vi "Tracker_hardware_setup.vi"(0 "VISA resource name":refnum<visa-resource-name>="ASRL3::INSTR", 2 "Close port? (T)":bool) -> (6 "error out":errorcluster, 7 "VISA resource name out":refnum<visa-resource-name>, 8 "ReadStatus":refnum<notifier>, 9 "error":bool, 10 "Record_flag":refnum<notifier>)   [LabVIEW 2016]
uses:
  <vilib>/Instr/_visa.llb/VISA Set IO Buffer Mask.ctl
  <vilib>/Instr/_visa.llb/VISA Configure Serial Port (Instr).vi
  Globaltracker.vi
panel:
  out "Poll Port data status":u32
  out "Port data status":i32
  out "error out 2":errorcluster
  out "read buffer":string
  out "Poll Binary":u32
  out "Poll Matrix":u32
  out "Poll Coord":u32
  out "Poll FPS":u32
  out "FPS status":i32
  out "Matrix mode status":string
  out "Coordinate mode status":string
  out "Binary mode status":string
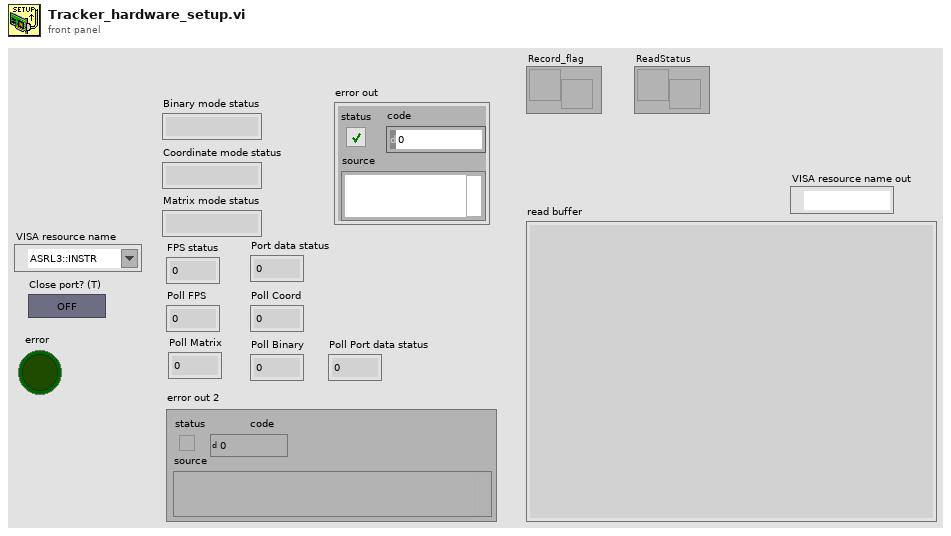
[diagram p1: front panel]
types:
  T1 = typedef "VISA Set IO Buffer Mask.ctl" = u16
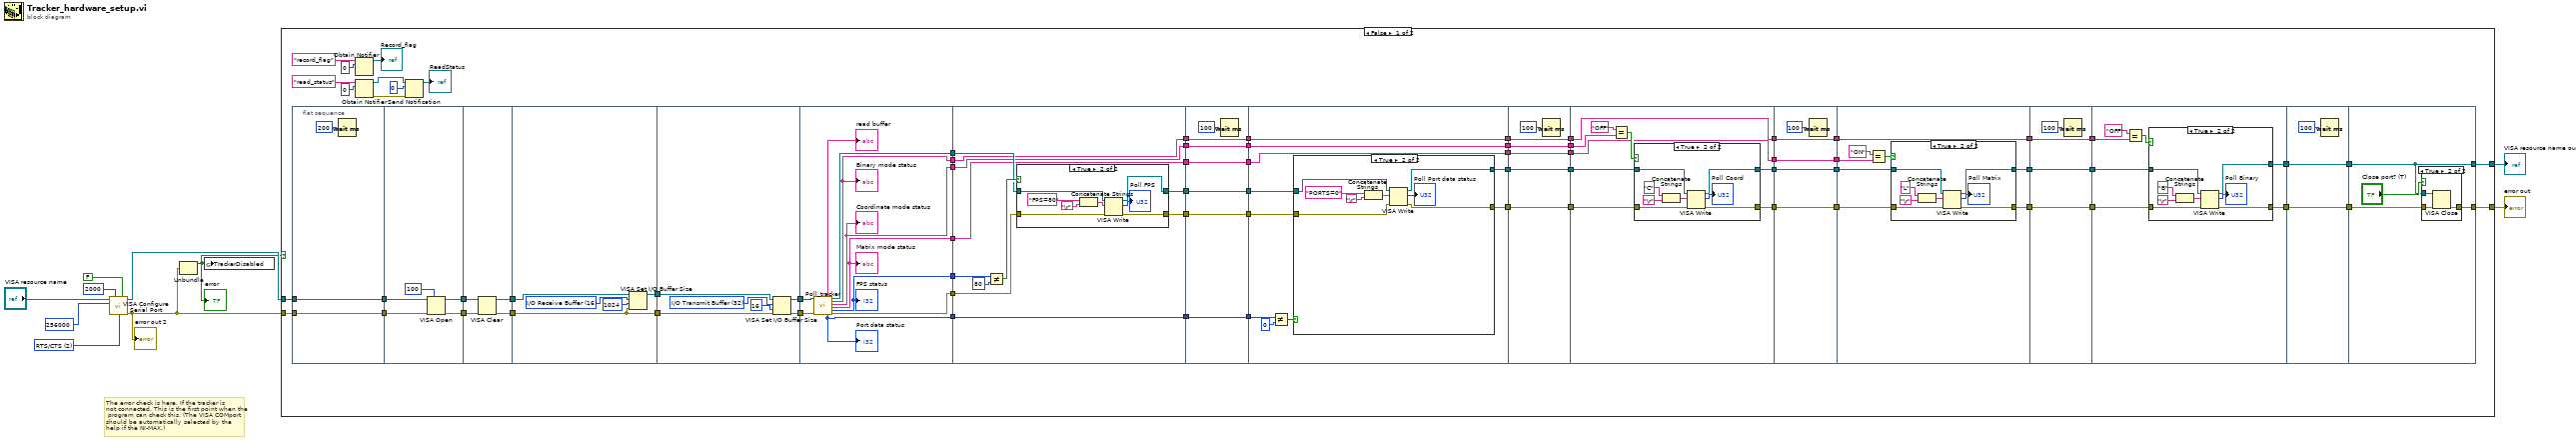
[diagram p0: block diagram]
diagram:
  w3 = u16 2 items=["None", "XON/XOFF", "RTS/CTS", "XON/XOFF & RTS/CTS", "DTR/DSR", "XON/XOFF & DTR/DSR"] ("flow control (0:none)")
  # "The error check is here. If the tracker is \nnot connected. This is the first point when the\n program can check this. (The VISA COMport \nshould be automatically selected by the \nhelp if the NI-MAX.)"
  n1 = call-poly "VISA Configure Serial Port"("VISA resource name"="VISA resource name", "timeout (10sec)"=u32 2000, "Enable Termination\nChar (T)"=FALSE ("Enable Termination\nChar (T)"), "baud rate (9600)"=u32 256000, "flow control (0:none)"=w3) -> ("VISA resource name out"=w6:refnum<visa-resource-name>, "error out"=w5:errorcluster)  [unwired: 9 in]
  "error out 2" <- w5
  n2 = Unbundle(w5) -> ("status"=w4:bool)  [unwired: 2 out]
  "error" <- w4
  n3 = global write "Globaltracker.vi" "TrackerDisabled"(w4) -> ()
  n4 = case shown="False" w4 {
    tunnel: w6 -> [w41 w242]
    tunnel: w5 -> [w40 w243]
    tunnel: [w12 w243] -> w2
    tunnel: [w11 w242] -> w1
    frame False {
      n5 = flat-sequence {
        tunnel: [w82] -> w80
        tunnel: [w81] -> w79
        tunnel: w41 -> [w82]
        tunnel: w40 -> [w81]
        tunnel: w80 -> [w86]
        tunnel: [w85] -> w77
        tunnel: w79 -> [w88]
        tunnel: [w87] -> w78
        tunnel: w78 -> [w91]
        tunnel: w77 -> [w92]
        tunnel: [w90] -> w76
        tunnel: [w89] -> w75
        tunnel: [w93] -> w73
        tunnel: [w97] -> w74
        tunnel: w76 -> [w93]
        tunnel: w75 -> [w95]
        tunnel: w74 -> [w101]
        tunnel: [w100] -> w72
        tunnel: w73 -> [w99]
        tunnel: [w98] -> w71
        tunnel: [w110] -> w69
        tunnel: [w111] -> w70
        tunnel: w72 -> [w113]
        tunnel: w71 -> [w112]
        tunnel: [w109] -> w68
        tunnel: [w108] -> w67
        tunnel: [w107] -> w66
        tunnel: [w106] -> w65
        tunnel: [w104] -> w30
        tunnel: w70 -> [w121]
        tunnel: [w118] -> w64
        tunnel: w69 -> [w120]
        tunnel: [w119] -> w63
        tunnel: w68 -> [w123]
        tunnel: [w117] -> w62
        tunnel: w67 -> [w117]
        tunnel: [w116] -> w61
        tunnel: w66 -> [w116]
        tunnel: [w115] -> w60
        tunnel: w65 -> [w115]
        tunnel: w30 -> [w114]
        tunnel: [w114] -> w13
        tunnel: w64 -> [w141]
        tunnel: [w141] -> w29
        tunnel: w63 -> [w140]
        tunnel: [w140] -> w28
        tunnel: [w138] -> w27
        tunnel: w62 -> [w138]
        tunnel: [w137] -> w26
        tunnel: w61 -> [w137]
        tunnel: [w136] -> w25
        tunnel: w60 -> [w136]
        tunnel: [w135] -> w14
        tunnel: w13 -> [w135]
        tunnel: w29 -> [w146]
        tunnel: [w145] -> w24
        tunnel: w28 -> [w148]
        tunnel: [w147] -> w22
        tunnel: w27 -> [w151]
        tunnel: [w151] -> w20
        tunnel: w26 -> [w150]
        tunnel: [w150] -> w18
        tunnel: w25 -> [w149]
        tunnel: [w149] -> w16
        tunnel: w14 -> [w143]
        tunnel: w24 -> [w167]
        tunnel: [w167] -> w23
        tunnel: w22 -> [w166]
        tunnel: [w166] -> w21
        tunnel: w20 -> [w165]
        tunnel: [w165] -> w19
        tunnel: w18 -> [w164]
        tunnel: [w164] -> w17
        tunnel: w16 -> [w163]
        tunnel: [w163] -> w15
        tunnel: w23 -> [w175]
        tunnel: [w173] -> w59
        tunnel: w21 -> [w174]
        tunnel: [w170] -> w58
        tunnel: w19 -> [w172]
        tunnel: w17 -> [w169]
        tunnel: [w169] -> w57
        tunnel: w15 -> [w168]
        tunnel: [w168] -> w56
        tunnel: w59 -> [w191]
        tunnel: [w191] -> w55
        tunnel: w58 -> [w190]
        tunnel: [w190] -> w54
        tunnel: [w188] -> w53
        tunnel: w57 -> [w188]
        tunnel: [w187] -> w52
        tunnel: w56 -> [w187]
        tunnel: w55 -> [w197]
        tunnel: [w195] -> w51
        tunnel: w54 -> [w196]
        tunnel: [w194] -> w50
        tunnel: w53 -> [w193]
        tunnel: w52 -> [w192]
        tunnel: [w192] -> w49
        tunnel: w51 -> [w213]
        tunnel: [w213] -> w48
        tunnel: w50 -> [w212]
        tunnel: [w212] -> w47
        tunnel: [w210] -> w46
        tunnel: w49 -> [w210]
        tunnel: w48 -> [w218]
        tunnel: [w216] -> w45
        tunnel: w47 -> [w217]
        tunnel: [w215] -> w44
        tunnel: w46 -> [w214]
        tunnel: w45 -> [w233]
        tunnel: [w233] -> w43
        tunnel: [w232] -> w42
        tunnel: w44 -> [w232]
        tunnel: w43 -> [w234]
        tunnel: w42 -> [w237]
        tunnel: [w235] -> w12
        tunnel: [w234] -> w11
        frame #0 {
          n6 = Wait (ms)(milliseconds to wait=u32 200) -> ()  [unwired: 1 out]
        }
        frame #1 {
          n7 = VISA Open(timeout (0)=u32 100 ("VISA Open timeout (0)"), error in (no error)=w88, VISA resource name=w86) -> (VISA resource name=w85:refnum<visa-resource-name>, error out=w87:errorcluster)  [unwired: 2 in]
        }
        frame #2 {
          n8 = VISA Clear(VISA resource name=w92, error in (no error)=w91) -> (VISA resource name out=w89:refnum<visa-resource-name>, error out=w90:errorcluster)
        }
        frame #3 {
          w94 = T1 16 items=["I/O Receive Buffer"=16, "I/O Transmit Buffer"=32, "I/O Receive and Transmit Buffer"=48] ("Mask")
          n9 = VISA Set I/O Buffer Size(VISA resource name=w95, mask (16)=w94, size (4096)=u32 1024, error in (no error)=w93) -> (VISA resource name out=w97:refnum<visa-resource-name>)  [unwired: 1 out]
        }
        frame #4 {
          w102 = T1 32 items=["I/O Receive Buffer"=16, "I/O Transmit Buffer"=32, "I/O Receive and Transmit Buffer"=48] ("Mask")
          n10 = VISA Set I/O Buffer Size(VISA resource name=w101, mask (16)=w102, size (4096)=u32 16, error in (no error)=w99) -> (VISA resource name out=w100:refnum<visa-resource-name>, error out=w98:errorcluster)
        }
        frame #5 {
          n11 = call "Poll_tracker.vi"("VISA resource name"=w113, "error in (no error)"=w112) -> ("read buffer"=→"read buffer":string, "Port data status"=w104:i32, "VISA resource name out"=w111:refnum<visa-resource-name>, "Binary mode status"=w106:string, "Coordinate mode status"=w108:string, "Matrix mode status"=w107:string, "FPS status"=w109:i32, "error out"=w110:errorcluster)  [unwired: 10 in]
          "Binary mode status" <- w106
          "Coordinate mode status" <- w108
          "Matrix mode status" <- w107
          "FPS status" <- w109
          "Port data status" <- w104
        }
        frame #6 {
          n12 = Not Equal?(x=w123, y=80) -> (x != y?=w124:bool)
          n13 = case shown="True" w124 {
            tunnel: w121 -> [w126 w130]
            tunnel: w120 -> [w125 w129]
            tunnel: [w125 w128] -> w119
            tunnel: [w126 w127] -> w118
            frame False {
            }
            frame True {
              n14 = Concatenate Strings("FPS=80" ("write buffer"), "\r") -> (w132:string)
              n15 = VISA Write(VISA resource name=w130, write buffer=w132, error in (no error)=w129) -> (VISA resource name out=w127:refnum<visa-resource-name>, return count=→"Poll FPS":u32, error out=w128:errorcluster)
            }
          }
        }
        frame #7 {
          n16 = Wait (ms)(milliseconds to wait=u32 100) -> ()  [unwired: 1 out]
        }
        frame #8 {
          n17 = Not Equal?(x=w143, y=0) -> (x != y?=w142:bool)
          n18 = case shown="True" w142 {
            tunnel: w148 -> [w152 w157]
            tunnel: [w152 w156] -> w147
            tunnel: w146 -> [w153 w155]
            tunnel: [w153 w154] -> w145
            frame False {
            }
            frame True {
              n19 = Concatenate Strings("PORTS=0" ("write buffer"), "\r") -> (w159:string)
              n20 = VISA Write(VISA resource name=w155, write buffer=w159, error in (no error)=w157) -> (VISA resource name out=w154:refnum<visa-resource-name>, return count=→"Poll Port data status":u32, error out=w156:errorcluster)
            }
          }
        }
        frame #9 {
          n21 = Wait (ms)(milliseconds to wait=u32 100) -> ()  [unwired: 1 out]
        }
        frame #10 {
          n22 = Equal?(x="OFF", y=w172) -> (x = y?=w176:bool)
          n23 = case shown="True" w176 {
            tunnel: w175 -> [w178 w182]
            tunnel: w174 -> [w177 w181]
            tunnel: [w178 w180] -> w173
            tunnel: [w177 w179] -> w170
            frame False {
            }
            frame True {
              n24 = Concatenate Strings("C" ("write buffer"), "\r") -> (w184:string)
              n25 = VISA Write(VISA resource name=w182, write buffer=w184, error in (no error)=w181) -> (VISA resource name out=w180:refnum<visa-resource-name>, return count=→"Poll Coord":u32, error out=w179:errorcluster)
            }
          }
        }
        frame #11 {
          n26 = Wait (ms)(milliseconds to wait=u32 100) -> ()  [unwired: 1 out]
        }
        frame #12 {
          n27 = Equal?(x="ON", y=w193) -> (x = y?=w199:bool)
          n28 = case shown="True" w199 {
            tunnel: w197 -> [w201 w205]
            tunnel: w196 -> [w200 w204]
            tunnel: [w201 w203] -> w195
            tunnel: [w200 w202] -> w194
            frame False {
            }
            frame True {
              n29 = Concatenate Strings("L" ("write buffer"), "\r") -> (w207:string)
              n30 = VISA Write(VISA resource name=w205, write buffer=w207, error in (no error)=w204) -> (VISA resource name out=w203:refnum<visa-resource-name>, return count=→"Poll Matrix":u32, error out=w202:errorcluster)
            }
          }
        }
        frame #13 {
          n31 = Wait (ms)(milliseconds to wait=u32 100) -> ()  [unwired: 1 out]
        }
        frame #14 {
          n32 = Equal?(x="OFF", y=w214) -> (x = y?=w220:bool)
          n33 = case shown="True" w220 {
            tunnel: w218 -> [w222 w226]
            tunnel: w217 -> [w221 w225]
            tunnel: [w222 w224] -> w216
            tunnel: [w221 w223] -> w215
            frame False {
            }
            frame True {
              n34 = Concatenate Strings("B" ("write buffer"), "\r") -> (w228:string)
              n35 = VISA Write(VISA resource name=w226, write buffer=w228, error in (no error)=w225) -> (VISA resource name out=w224:refnum<visa-resource-name>, return count=→"Poll Binary":u32, error out=w223:errorcluster)
            }
          }
        }
        frame #15 {
          n36 = Wait (ms)(milliseconds to wait=u32 100) -> ()  [unwired: 1 out]
        }
        frame #16 {
          n37 = case shown="True" "Close port? (T)" {
            tunnel: w237 -> [w238 w241]
            tunnel: [w238 w240] -> w235
            tunnel: w234 -> [_ w239]
            frame False {
            }
            frame True {
              n38 = VISA Close(VISA resource name=w239, error in (no error)=w241) -> (error out=w240:errorcluster)
            }
          }
        }
      }
      n39 = Obtain Notifier(name (unnamed)="record_flag", notification data type=0) -> (notifier out=→"Record_flag":refnum<notifier>)  [unwired: 2 in, 2 out]
      n40 = Obtain Notifier(name (unnamed)="read_status", notification data type=0) -> (notifier out=w35:refnum<notifier>, error out=w36:errorcluster)  [unwired: 2 in, 1 out]
      n41 = Send Notification(notification=0, notifier=w35, error in (no error)=w36) -> (notifier out=→"ReadStatus":refnum<notifier>)  [unwired: 1 out]
    }
    frame True {
    }
  }
  "error out" <- w2
  "VISA resource name out" <- w1
